vi "UpdateAnalysisName.vi"() -> ()   [LabVIEW 2015]
uses:
  Process/Controls/Process_Type.ctl
  Process/Controls/Process_Setting.ctl
  Control/CoordinateAnalysisSetting.ctl
  Caliper/Controls/CaliperType.ctl
  Caliper/Controls/SelectionListEntryPointType.ctl
  Caliper/Controls/SelectionListEntry.ctl
  Caliper/Controls/CaliperResult.ctl
  Caliper/Controls/CaliperDataEntry.ctl
  Control/CoordinateCaliperSetting.ctl
  Control/CoordinatteEntry.ctl
panel:
  in  "CoordinatteEntry":T1 {"CaliperSetting"."CaliperEntry"."CaliperType" items=["Distance", "Mid Point", "Perpendicular Projection", "Lines Intersection", "Angle from Horizontal", "Angle from Vertical", "Angle Defined by 3 Points", "Angle Defined by 4 Points", "Bissecting Line", "Mid Line", "Center of Mass", "Area", "Line Fit", "Circle Fit", "Ellipse Fit"]; "OriginPointInfo"."Mode" items=["Horizontal Motion", "Vertical Motion", "Horizontal and Vertical Motion", "Horizontal. Vertical and Angular Motion"]; "AnalysisSetting"."ROI"."Contours"."Type" items=["No Selection", "Point", "Line", "Rectangle", "Oval", "Polygon", "Freehand Region", "Annulus", "Unused2", "Unused3", "Broken Line", "Freehand Line", "Rotated Rectangle"]}
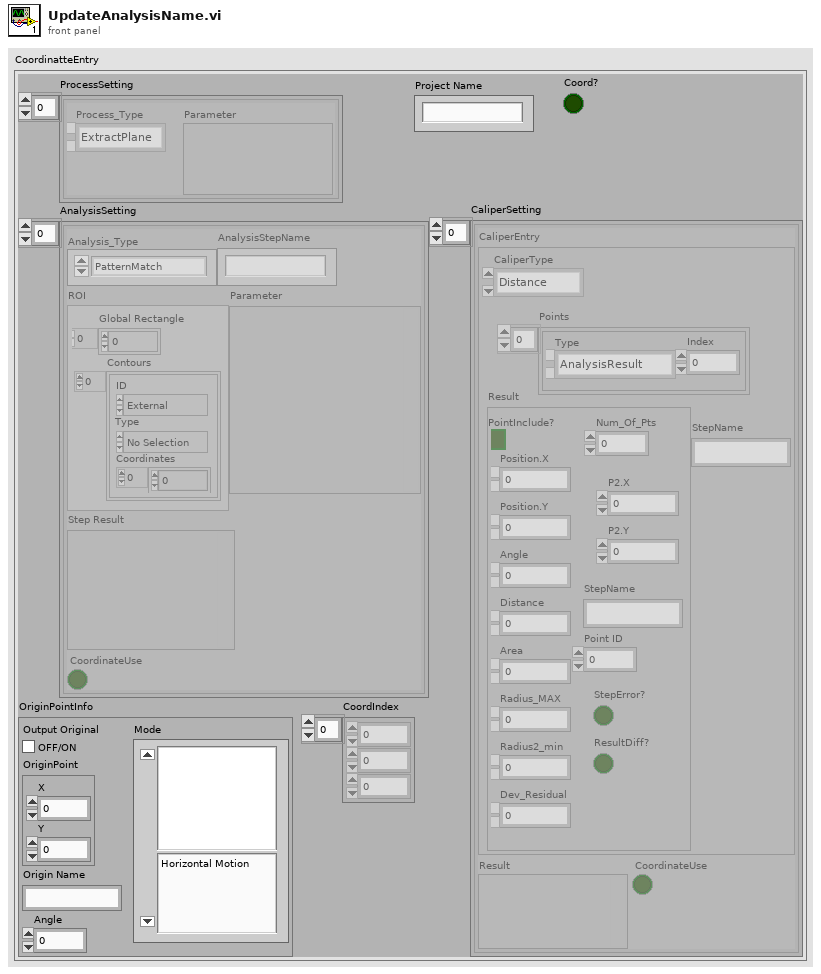
[diagram p1: front panel]
types:
  T1 = typedef "CoordinatteEntry.ctl" = cluster{"ProcessSetting":T2[], "Project Name":string, "AnalysisSetting":T4[], "Coord?":bool, "OriginPointInfo":cluster{"Output Original":bool, "Origin Name":string, "Angle":dbl, "Mode":u16, "OriginPoint":cluster{"X":dbl, "Y":dbl}}, "CaliperSetting":T6[], "CoordIndex":i32[]}
  T2 = typedef "Process_Setting.ctl" = cluster{"Process_Type":T3, "Parameter":variant}
  T3 = typedef "Process_Type.ctl" = enum16{"None", "ExtractPlane", "BinaryMono", "Operators", "GrayMorphology", "Filters", "Lookup Table", "Particle Filter", "Mask"}
  T4 = typedef "CoordinateAnalysisSetting.ctl" = cluster{"Analysis_Type":enum16{"PatternMatch", "Straight Edge"}, "ROI ":T5, "Parameter":variant, "Step Result":variant, "AnalysisStepName":string, "CoordinateUse":bool}
  T5 = typedef "ROI Descriptor" = cluster{"Global Rectangle":i32[], "Contours":cluster{"ID":enum32{"External", "Internal"}, "Type":u32, "Coordinates":i32[]}[]}
  T6 = typedef "CoordinateCaliperSetting.ctl" = cluster{"Result":variant, "CoordinateUse":bool, "CaliperEntry":T7}
  T7 = typedef "CaliperDataEntry.ctl" = cluster{"CaliperType":T8, "Points":T9[], "Result":T11, "StepName":string}
  T8 = typedef "CaliperType.ctl" = u32
  T9 = typedef "SelectionListEntry.ctl" = cluster{"Type":T10, "Index":i32}
  T10 = typedef "SelectionListEntryPointType.ctl" = enum16{"AnalysisResult", "CaliperResult"}
  T11 = typedef "CaliperResult.ctl" = cluster{"PointInclude?":bool, "Num_Of_Pts":u8, "Position.X":dbl, "Position.Y":dbl, "Angle":dbl, "Distance":dbl, "Area":dbl, "Radius_MAX":dbl, "Radius2_min":dbl, "Dev_Residual":dbl, "P2.X":dbl, "P2.Y":dbl, "StepName":string, "Point ID":u8, "StepError?":bool, "ResultDiff?":bool}
  T12 = cluster{"Point1 (Pixels)":cluster{"X":sgl, "Y":sgl}, "Point2 (Pixels)":cluster{"X":sgl, "Y":sgl}, "Point1 (Real-World)":cluster{"X":sgl, "Y":sgl}, "Point2 (Real-World)":cluster{"X":sgl, "Y":sgl}, "Angle (Pixel)":dbl, "Angle (Real-World)":dbl, "Score":dbl, "Straightness":dbl, "Average SNR (db)":dbl, "Calibration Valid":bool}[]
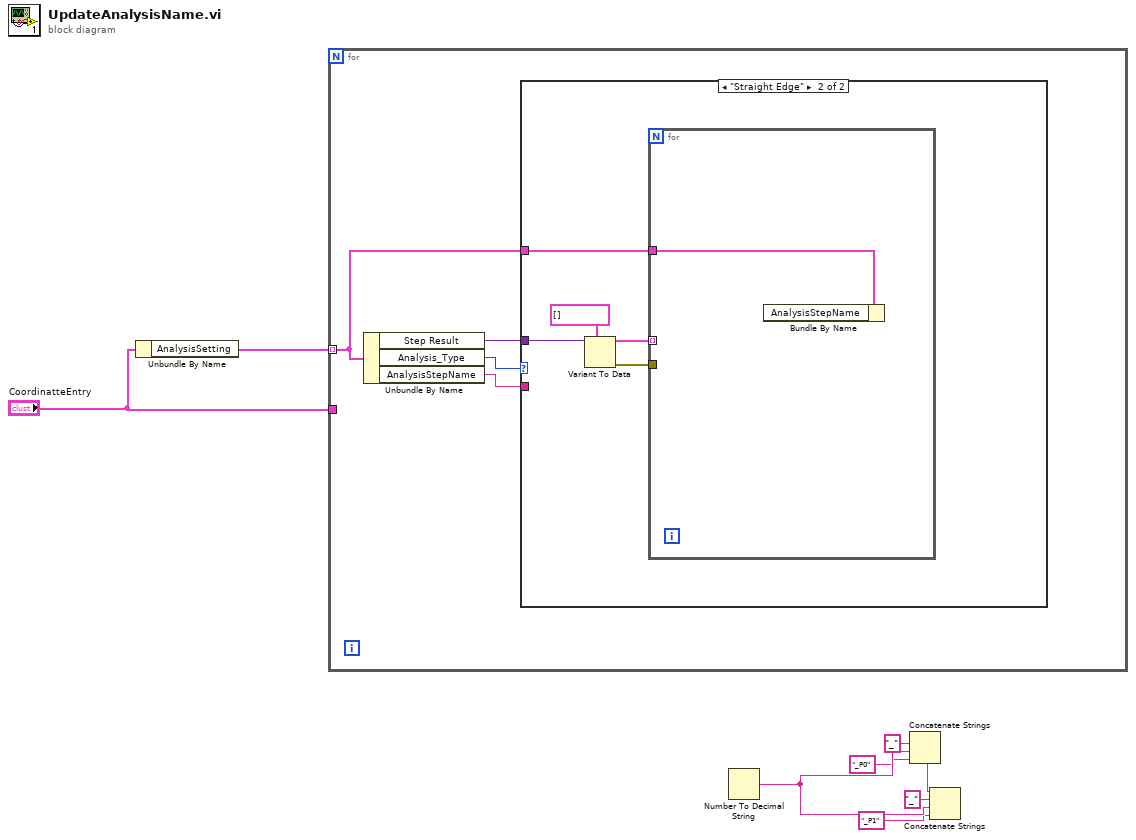
[diagram p0: block diagram]
diagram:
  n1 = Unbundle By Name("CoordinatteEntry") -> ("AnalysisSetting"=w8:T4[])
  n2 = for {
    tunnel: w8 -> [w12] mode=indexing
    tunnel: "CoordinatteEntry" -> [_]
    n3 = Unbundle By Name(w12) -> ("Step Result"=w11:variant, "Analysis_Type"=w10:enum16{"PatternMatch", "Straight Edge"}, "AnalysisStepName"=w9:string)
    n4 = case shown="\"Straight Edge\"" w10 {
      tunnel: w12 -> [_ w14]
      tunnel: w11 -> [_ w13]
      tunnel: w9 -> [_ _]
      frame "PatternMatch", Default {
      }
      frame "Straight Edge" {
        n5 = Variant To Data(type=T12 [] ("Straight Edge Cluster Array"), Variant=w13) -> (data=w17:T12, error out=w16:errorcluster)  [unwired: 1 in]
        n6 = for {
          tunnel: w17 -> [_] mode=indexing
          tunnel: w16 -> [_]
          tunnel: w14 -> [w18]
          n7 = Bundle By Name(cluster=w18) -> ()  [unwired: 1 in, 1 out]
        }
      }
    }
  }
  n8 = Number To Decimal String() -> (decimal integer string=w5:string)  [unwired: 2 in]
  n9 = Concatenate Strings("_" ("string"), w5, "_P0" ("string")) -> (w6:string)  [unwired: 1 out]
  n10 = Concatenate Strings(w6, "_" ("string"), w5, "_P1" ("string")) -> ()  [unwired: 1 out]
